vi "CRYDelete Complete From Step.vi"(10 "Step No.":i32[](array[numeric]), 11 "Type In":T1(ring)) -> (3 "Step No out":i32[](array[numeric]))   [LabVIEW 2013]
uses:
  CRYSystem/Task Sequence/CRYProject Run Control Global.vi
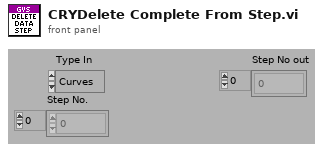
[diagram p1: front panel]
types:
  T1 = enum16{"Curves", "Values", "Results", "WFM", "All"}
  T2 = enum16{"Curves", "Values", "Results", "WFM", "All"}[]
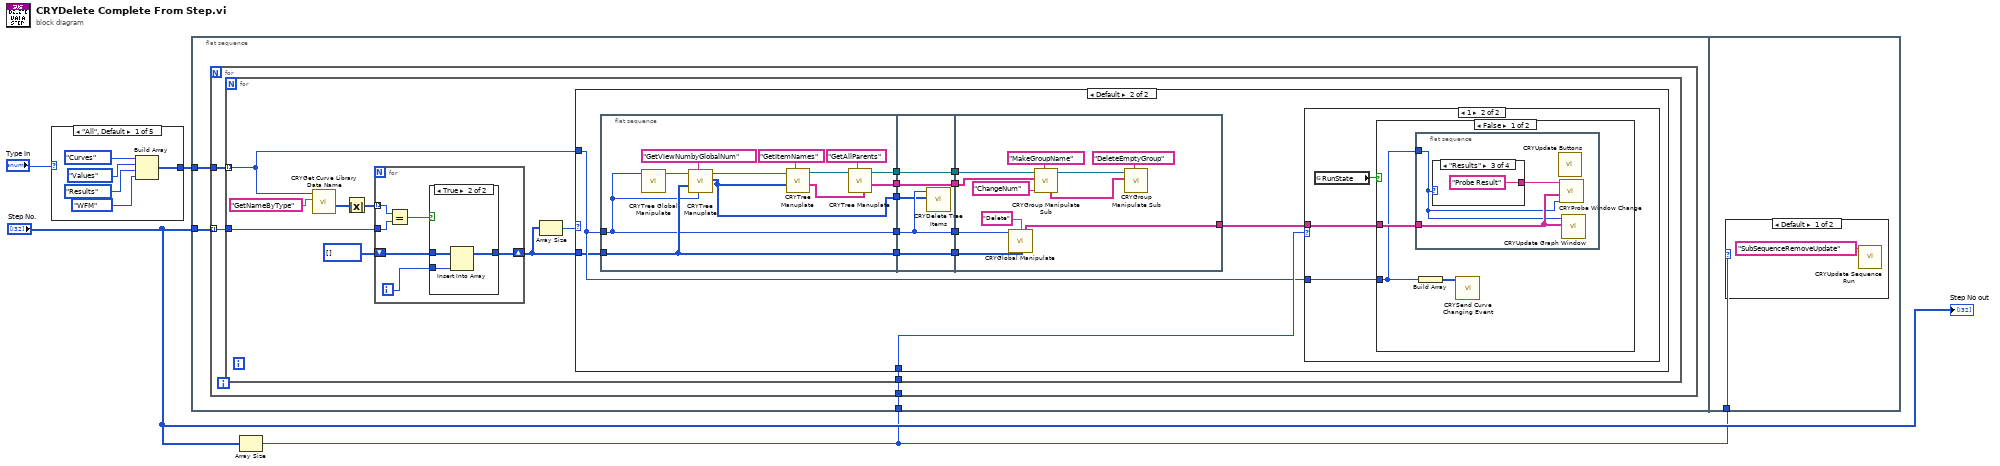
[diagram p0: block diagram]
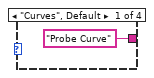
[diagram p5: hidden frame]
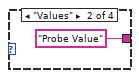
[diagram p6: hidden frame]
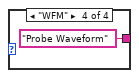
[diagram p7: hidden frame]
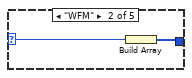
[diagram p10: hidden frame]
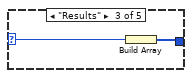
[diagram p11: hidden frame]
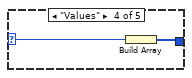
[diagram p12: hidden frame]
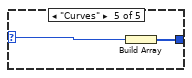
[diagram p13: hidden frame]
diagram:
  n1 = case shown="\"All\", Default" "Type In" {
    selector: "Type In" -> [_ w10 w12 w14 w16]
    tunnel: [w8 w11 w13 w15 w17] -> w3
    frame "All", Default {
      n2 = Build Array(enum16{"Curves", "Values", "Results", "WFM"}."Curves" ("Type"), enum16{"Curves", "Values", "Results", "WFM"}."Values" ("Type"), enum16{"Curves", "Values", "Results", "WFM"}."Results" ("Type"), enum16{"Curves", "Values", "Results", "WFM"}."WFM" ("Type")) -> (w8:enum16{"Curves", "Values", "Results", "WFM"}[])
    }
    frame "WFM" {
      n3 = Build Array(w10) -> (w11:T2)
    }
    frame "Results" {
      n4 = Build Array(w12) -> (w13:T2)
    }
    frame "Values" {
      n5 = Build Array(w14) -> (w15:T2)
    }
    frame "Curves" {
      n6 = Build Array(w16) -> (w17:T2)
    }
  }
  n7 = flat-sequence {
    tunnel: w3 -> [w20]
    tunnel: "Step No." -> [w19]
    tunnel: w1 -> [w18]
    tunnel: w1 -> [w97]
    frame #0 {
      n8 = for {
        tunnel: w20 -> [w23]
        tunnel: w19 -> [w22] mode=indexing
        tunnel: w18 -> [w21]
        n9 = for {
          tunnel: w22 -> [w32]
          tunnel: w23 -> [w31] mode=indexing
          tunnel: w21 -> [w30]
          n10 = call "CRYGet Curve Library Data Name.vi"("sAction"="GetNameByType", "Type"=w31) -> ("nStep No"=w27:i32[])  [unwired: 4 in, 5 out]
          n11 = Absolute Value(x=w27) -> (abs(x)=w24:i32[])
          n12 = for {
            tunnel: w32 -> [w36]
            tunnel: w24 -> [w37] mode=indexing
            shift-right: [w34] -> w29
            shift-left: i32[] [] ("Step No.") -> [w35]
            i -> [w33]
            n13 = Equal?(x=w37, y=w36) -> (x = y?=w38:bool)
            n14 = case shown="True" w38 {
              tunnel: [w39 w41] -> w34
              tunnel: w35 -> [w39 w42]
              tunnel: w33 -> [_ w40]
              frame False {
              }
              frame True {
                n15 = Insert Into Array(array=w42, new element=w40) -> (w41:i32[])  [unwired: 1 in]
              }
            }
          }
          n16 = Array Size(array=w29) -> (size(s)=w28:i32)
          n17 = case shown="Default" w28 {
            tunnel: w31 -> [_ w54]
            tunnel: w30 -> [_ w55]
            tunnel: w29 -> [_ w52]
            frame 0 {
            }
            frame Default {
              n18 = flat-sequence {
                tunnel: w52 -> [w65]
                tunnel: w54 -> [w64]
                tunnel: [w64] -> w51
                tunnel: [w65] -> w49
                tunnel: [w58] -> w47
                tunnel: [w57] -> w46
                tunnel: [w56] -> w43
                tunnel: w51 -> [w71]
                tunnel: [w71] -> w50
                tunnel: w49 -> [w72]
                tunnel: [w72] -> w48
                tunnel: w47 -> [w70]
                tunnel: w46 -> [w69]
                tunnel: [w69] -> w45
                tunnel: [w68] -> w44
                tunnel: w43 -> [w68]
                tunnel: [w81] -> w53
                tunnel: w50 -> [w82]
                tunnel: w48 -> [w80]
                tunnel: w45 -> [w77]
                tunnel: w44 -> [w74]
                frame #0 {
                  n19 = call "CRYTree Global Manipulate.vi"("Type In"=w64) -> ("Tree/Curve Tree"=w66:refnum<vi>)  [unwired: 7 in, 3 out]
                  n20 = call "CRYTree Manuplate.vi"("Type"=w64, "sAction"="GetViewNumbyGlobalNum", "nData"=w65, "Tree in"=w66) -> ("nData Out"=w58:i32[], "Tree Out"=w59:refnum<vi>)  [unwired: 4 in, 2 out]
                  n21 = call "CRYTree Manuplate.vi"("sAction"="GetItemNames", "nData"=w58, "Tree in"=w59) -> ("sData Out"=w63:string[], "Tree Out"=w62:refnum<vi>)  [unwired: 5 in, 2 out]
                  n22 = call "CRYTree Manuplate.vi"("sData"=w63, "sAction"="GetAllParents", "Tree in"=w62) -> ("sData Out"=w56:string[], "Tree Out"=w57:refnum<vi>)  [unwired: 5 in, 2 out]
                }
                frame #1 {
                  n23 = call "CRYDelete Tree Items.vi"("Array"=w70, "Type"=w71) -> ()  [unwired: 2 in, 8 out]
                }
                frame #2 {
                  n24 = call "CRYGlobal Manipulate.vi"("Type"=w82, "sAction"="Delete", "nData"=w80) -> ("sData Out"=w81:string[])  [unwired: 6 in, 6 out]
                  n25 = call "CRYGroup Manipulate Sub.vi"("sAction"="MakeGroupName", "sOption"="ChangeNum", "sData"=w74, "Tree in"=w77) -> ("Tree Out"=w75:refnum<vi>, "sData Out"=w73:string[])  [unwired: 3 in, 3 out]
                  n26 = call "CRYGroup Manipulate Sub.vi"("sAction"="DeleteEmptyGroup", "sData"=w73, "Tree in"=w75) -> ()  [unwired: 4 in, 5 out]
                }
              }
              n27 = case shown="1" w55 {
                tunnel: w54 -> [_ w86]
                tunnel: w53 -> [_ w85]
                frame Default {
                  # "in the case of SubSequenceRemoveUpdate."
                }
                frame 1 {
                  n28 = global read "CRYProject Run Control Global.vi" "RunState"() -> (w84:bool)
                  n29 = case shown="False" w84 {
                    tunnel: w86 -> [w87 _]
                    tunnel: w85 -> [w89 _]
                    frame False {
                      n30 = flat-sequence {
                        tunnel: w89 -> [w91]
                        tunnel: w87 -> [w90]
                        frame #0 {
                          n31 = case shown="\"Results\"" w90 {
                            tunnel: ["Probe Curve" "Probe Value" "Probe Result" "Probe Waveform"] -> w92
                            frame "Curves", Default {
                            }
                            frame "Values" {
                            }
                            frame "Results" {
                            }
                            frame "WFM" {
                            }
                          }
                          n32 = call "CRYUpdate Buttons.vi"() -> ()  [unwired: 1 in, 11 out]
                          n33 = call "CRYProbe Window Change.vi"("Type"=w90, "Close Names"=w91, "Probe Type"=w92) -> ()  [unwired: 2 in, 7 out]
                          n34 = call "CRYUpdate Graph Window.vi"("Del/Update Names"=w91, "Type"=w90) -> ()  [unwired: 3 in, 7 out]
                        }
                      }
                      n35 = Build Array(w87) -> (w88:T2)
                      n36 = call "CRYSend Curve Changing Event.vi"("Type"=w88) -> ()  [unwired: 11 out]
                    }
                    frame True {
                    }
                  }
                }
              }
            }
          }
        }
      }
    }
    frame #1 {
      n37 = case shown="Default" w97 {
        frame Default {
          n38 = call "CRYUpdate Sequence Run.vi"("sOption"="SubSequenceRemoveUpdate") -> ()  [unwired: 11 in]
        }
        frame 1 {
        }
      }
    }
  }
  n39 = Array Size(array="Step No.") -> (size(s)=w1:i32)
  "Step No out" <- "Step No."
